vi "LIBRARY PROJECT.vi"() -> ()   [LabVIEW 2016]
panel:
  out "?":string
  out "?":string
  out "?":string
  in  "ROLL.NO":i32
  in  "?":bool
  # "DEPARTMENT OF ELECTRONICS AND INSTRUMENTATION"
  # "LIBRARY  BOOKS  DATA"
  # "DETAILS"
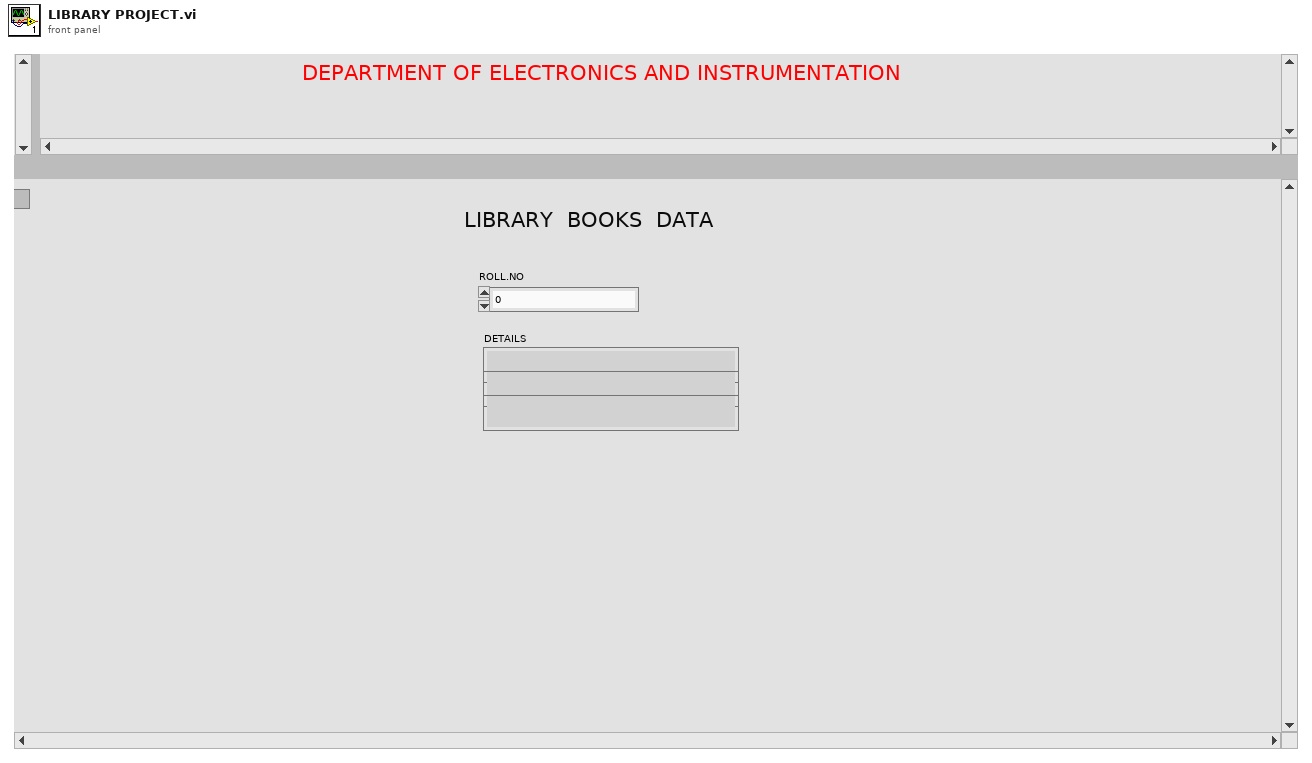
[diagram p1: front panel]
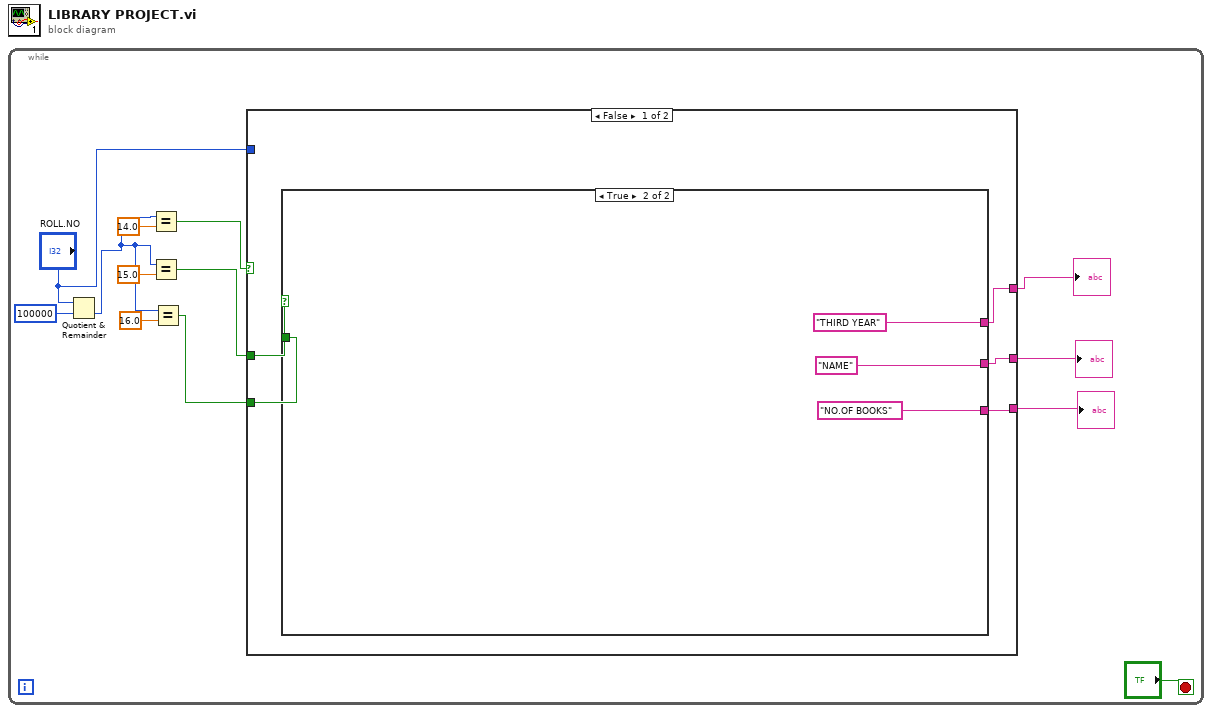
[diagram p0: block diagram]
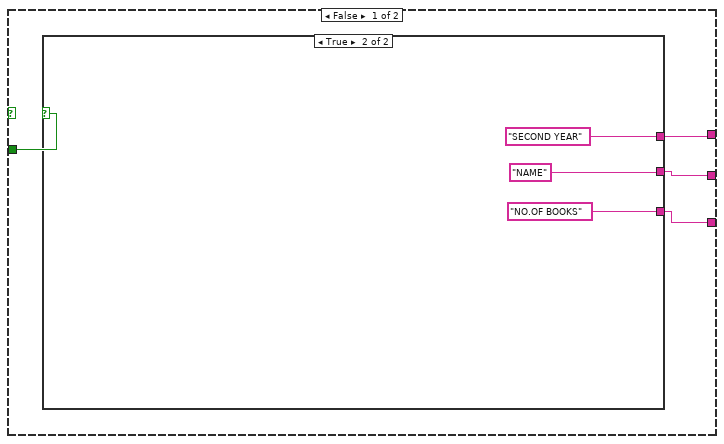
[diagram p2: hidden frame]
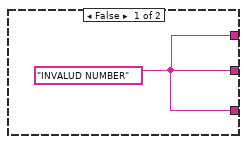
[diagram p3: hidden frame]
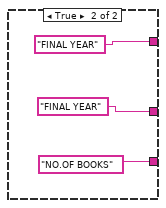
[diagram p4: hidden frame]
diagram:
  n1 = while {
    stop <- "?" stop-if-true
    n2 = Quotient & Remainder(x="ROLL.NO", y=100000) -> (floor(x/y)=w2:i32)  [unwired: 1 out]
    n3 = Equal?(x=w2, y=14.0) -> (x = y?=w10:bool)
    n4 = Equal?(x=w2, y=15.0) -> (x = y?=w9:bool)
    n5 = Equal?(x=w2, y=16.0) -> (x = y?=w8:bool)
    n6 = case shown="False" w10 {
      tunnel: w9 -> [w18 _]
      tunnel: w8 -> [w17 _]
      tunnel: [w16 "FINAL YEAR"] -> w7
      tunnel: [w15 "FINAL YEAR"] -> w6
      tunnel: [w14 "NO.OF BOOKS"] -> w5
      tunnel: "ROLL.NO" -> [_ _]
      frame False {
        n7 = case shown="True" w18 {
          tunnel: w17 -> [w22 _]
          tunnel: [w21 "THIRD YEAR"] -> w16
          tunnel: [w20 "NAME"] -> w15
          tunnel: [w19 "NO.OF BOOKS"] -> w14
          frame False {
            n8 = case shown="True" w22 {
              tunnel: [w23 "SECOND YEAR"] -> w21
              tunnel: [w23 "NAME"] -> w20
              tunnel: [w23 "NO.OF BOOKS"] -> w19
              frame False {
                w23 = "INVALUD NUMBER"
              }
              frame True {
              }
            }
          }
          frame True {
          }
        }
      }
      frame True {
      }
    }
    "?" <- w6
    "?" <- w7
    "?" <- w5
  }
